vi "Unflatten.vi"(8 "error in (no error)":errorcluster, 10 "JSON stream":string, 11 "JSON Object In":refnum<class "JSON Object.lvclass">) -> (0 "error out":errorcluster, 1 "Empty?":bool, 2 "rest of JSON stream":string, 3 "JSON Object Out":refnum<class "JSON Object.lvclass">)   [LabVIEW 2011, in "JSON Object.lvclass"]
uses:
  JSON Object.lvclass
  JSON Value/JSON Value.lvclass
  JSON Object.lvclass/JSON Object.ctl
  JSON Scalar/Parse In String.vi
  JSON Scalar/Strip Quotes.vi
  JSON Scalar/Unescape JSON string.vi
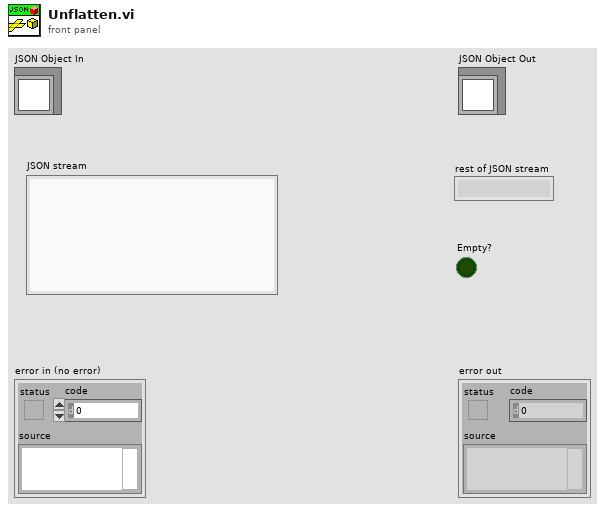
[diagram p1: front panel]
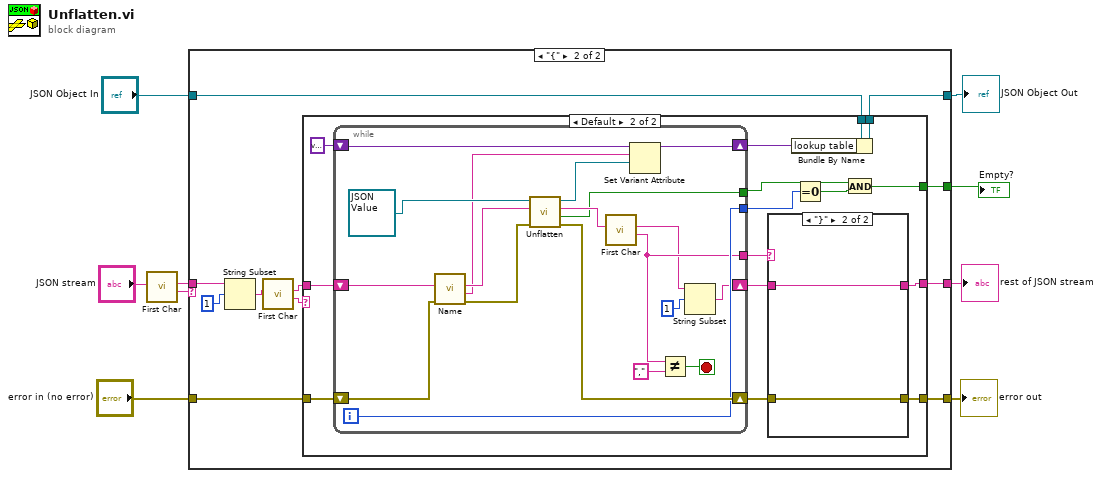
[diagram p0: block diagram]
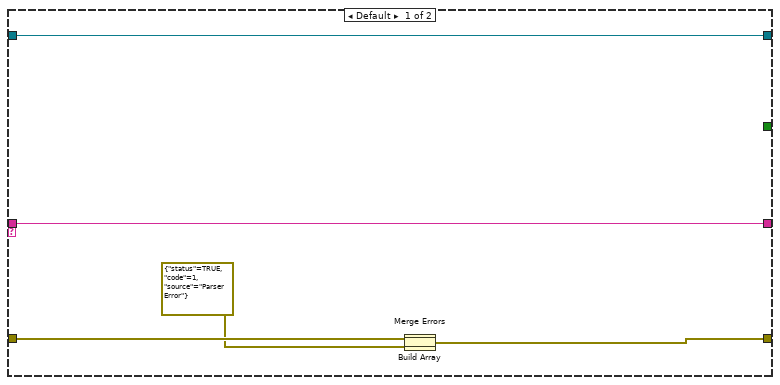
[diagram p2: hidden frame]
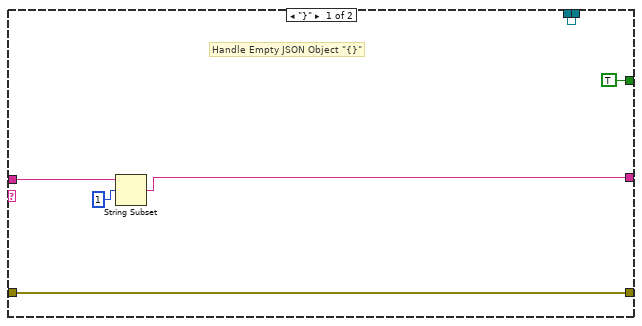
[diagram p3: hidden frame]
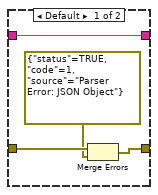
[diagram p4: hidden frame]
diagram:
  n1 = call "First Char.vi"("String in"="JSON stream") -> ("First Char"=w8:string, "String"=w7:string)  [unwired: 9 in]
  n2 = case shown="\"{\"" w8 {
    tunnel: w7 -> [w12 w19]
    tunnel: [w14 w22] -> w6
    tunnel: "error in (no error)" -> [w15 w24]
    tunnel: [w12 w23] -> w4
    tunnel: [w11 w25] -> w3
    tunnel: "JSON Object In" -> [w11 w26]
    tunnel: [_ w21] -> w1
    frame Default {
      n3 = Build Array(w15, errorcluster {"status"=TRUE, "code"=1, "source"="Parser Error"} ("error in")) -> (w10:errorcluster[])
      n4 = Merge Errors(w10) -> (w14:errorcluster)
    }
    frame "{" {
      n5 = String Subset(string=w19, offset (0)=1 ("length (rest)")) -> (substring=w17:string)  [unwired: 1 in]
      n6 = call "First Char.vi"("String in"=w17) -> ("First Char"=w16:string, "String"=w18:string)  [unwired: 9 in]
      n7 = case shown="Default" w16 {
        tunnel: w18 -> [w28 w47]
        tunnel: w26 -> [w32 w46]
        tunnel: [w32 w45] -> w25
        tunnel: w24 -> [w30 w44]
        tunnel: [w27 w42] -> w23
        tunnel: [w30 w40] -> w22
        tunnel: [TRUE w33] -> w21
        frame "}" {
          # "Handle Empty JSON Object \"{}\""
          n8 = String Subset(string=w28, offset (0)=1 ("length (rest)")) -> (substring=w27:string)  [unwired: 1 in]
        }
        frame Default {
          n9 = while {
            shift-right: [w54] -> w43
            shift-left: w47 -> [w58]
            tunnel: [w57] -> w41
            shift-right: [w69] -> w39
            shift-left: w44 -> [w60]
            shift-right: [w64] -> w37
            shift-left: variant -> [w63]
            tunnel: [w62] -> w35
            tunnel: [w61] -> w36
            i -> [w61]
            stop <- w70 stop-if-true
            n10 = call "Name.vi"("error in (no error)"=w60, "String in"=w58) -> ("error out"=w59:errorcluster, "JSON name"=w66:string, "Rest of string"=w67:string)  [unwired: 7 in]
            n11 = call-dynamic "Unflatten.vi"("error in (no error)"=w59, "JSON stream"=w67, "JSON Value in"=refnum<class "JSON Value.lvclass"> refnum ("JSON Value.lvclass")) -> ("error out"=w69:errorcluster, "Empty?"=w62:bool, "rest of JSON stream"=w72:string, "JSON Value out"=w65:refnum<class "JSON Value.lvclass">)  [unwired: 5 in]
            n12 = call "First Char.vi"("String in"=w72) -> ("First Char"=w57:string, "String"=w55:string)  [unwired: 9 in]
            n13 = Set Variant Attribute(Variant=w63, name=w66, value=w65) -> (Variant out=w64:variant)  [unwired: 1 in, 2 out]
            n14 = Not Equal?(x=w57, y=",") -> (x != y?=w70:bool)
            n15 = String Subset(string=w55, offset (0)=1 ("length (rest)")) -> (substring=w54:string)  [unwired: 1 in]
          }
          n16 = case shown="\"}\"" w41 {
            tunnel: w43 -> [w50 w52]
            tunnel: [w50 w52] -> w42
            tunnel: [w51 w53] -> w40
            tunnel: w39 -> [w49 w53]
            frame Default {
              n17 = Merge Errors(w49, errorcluster {"status"=TRUE, "code"=1, "source"="Parser Error: JSON Object"} ("error in")) -> (w51:errorcluster)
            }
            frame "}" {
            }
          }
          n18 = Bundle By Name(cluster=w46, "lookup table"=w37) -> (w45:refnum<class "JSON Object.lvclass">)
          n19 = Equal To 0?(x=w36) -> (x = 0?=w34:bool)
          n20 = And(x=w35, y=w34) -> (x .and. y?=w33:bool)
        }
      }
    }
  }
  "error out" <- w6
  "JSON Object Out" <- w3
  "rest of JSON stream" <- w4
  "Empty?" <- w1
